vi "Get Cluster Elements (data types).vi"(8 "Error In":errorcluster, 9 "Type In":variant, 10 "Cluster":variant, 11 "Type Enum (Cluster)":T1=enum."Cluster") -> (0 "Error Out":errorcluster, 1 "Types Out":variant[](array[variant]), 2 "Cluster Elements":variant[](array[variant]))   [LabVIEW 2020]
doc: "This VI was created for use with the Read/Write Cluster VIs. It breaks a cluster up into its individual elements and passes the elements out in an array of variants.\n\nFreeware from Moore Good Ideas, www.mooregoodideas.com. Do not remove this line."
uses:
  <vilib>/Utility/VariantDataType/Type.ctl
  <vilib>/Utility/Data Type/NI_Data Type.lvlib
  <vilib>/Utility/VariantDataType/VariantType.lvlib
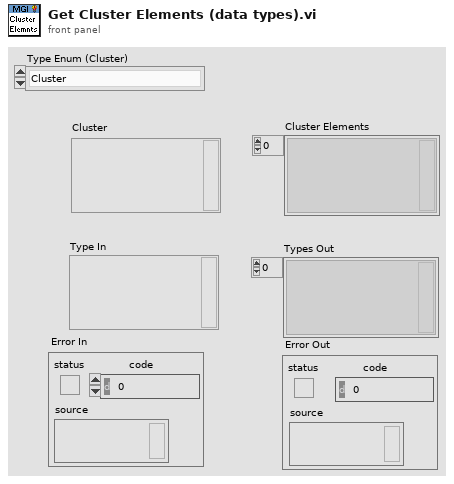
[diagram p1: front panel]
types:
  T1 = typedef "VariantType.lvlib/Type.ctl" = enum8{"Invalid Type", "Void", "I8", "I16", "I32", "I64", "U8", "U16", "U32", "U64", "Single Float", "Double Float", "Extended Float", "Single Complex", "Double Complex", "Extended Complex", "Enum U8", "Enum U16", "Enum U32", "Enum U64", "Single Float With Unit", "Double Float With Unit", "Extended Float With Unit", "Single Complex with Unit", "Double Complex with Unit", "Extended Complex with Unit", "Boolean", "String", "Path", "Picture", "Tag", "Array", "Cluster", "Variant", "LV Variant", "Waveform", "Timestamp", "Digital Waveform", "Digital Data", "ExpressData", "Refnum", "External Data", "VI", "Poly VI", "LabVIEW Class Instance", "Fixed Point"}
  T2 = typedef "NI_Data Type.lvlib/Data Type.ctl" = enum8{"Invalid Type", "Void", "I8", "I16", "I32", "I64", "U8", "U16", "U32", "U64", "Single Float", "Double Float", "Extended Float", "Single Complex", "Double Complex", "Extended Complex", "Enum U8", "Enum U16", "Enum U32", "Enum U64", "Single Float With Unit", "Double Float With Unit", "Extended Float With Unit", "Single Complex with Unit", "Double Complex with Unit", "Extended Complex with Unit", "Boolean", "String", "Path", "Picture", "Tag", "Array", "Cluster", "Variant", "LV Variant", "Waveform", "Timestamp", "Digital Waveform", "Digital Data", "ExpressData", "Refnum", "External Data", "VI", "Poly VI", "LabVIEW Class Instance", "Fixed Point", "Set Collection", "Map Collection"}
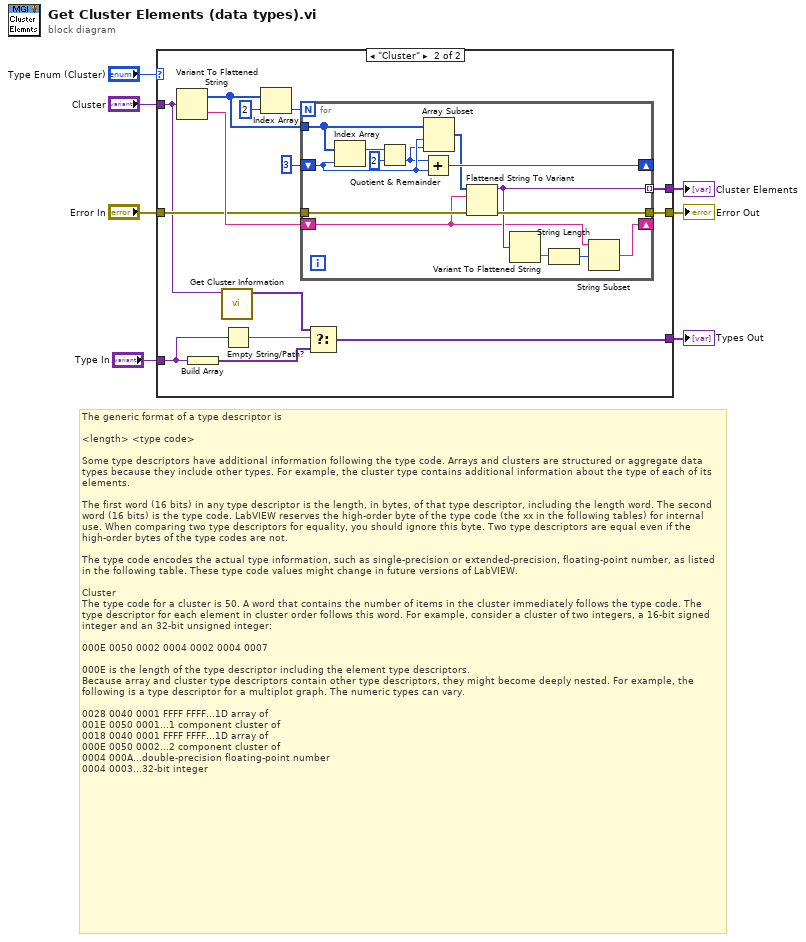
[diagram p0: block diagram]
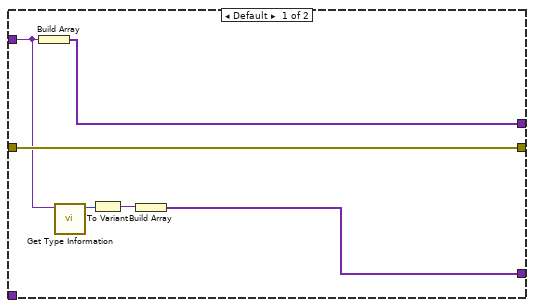
[diagram p2: hidden frame]
diagram:
  # "The generic format of a type descriptor is\n\n<length> <type code> \n\nSome type descriptors have additional information following the type code. Arrays and clusters are structured or aggregate data types because they include other types. For example, the cluster type contains additional information about the type of each of its elements.\n\nThe first word (16 bits) in any type descriptor is the length, in bytes, of that type descriptor, including the length word. The second word (16 bits) is the type code. LabVIEW reserves the high-order byte of the type code (the xx in the following tables) for internal use. When comparing two type descriptors for equality, you should ignore this byte. Two type descriptors are equal even if the high-order bytes of the type codes are not.\n\nThe type code encodes the actual type information, such as single-precision or extended-precision, floating-point number, as listed in the following table. These type code values might change in future versions of LabVIEW.\n\nCluster\nThe type code for a cluster is 50. A word that contains the number of items in the cluster immediately follows the type code. The type descriptor for each element in cluster order follows this word. For example, consider a cluster of two integers, a 16-bit signed integer and an 32-bit unsigned integer:\n\n000E 0050 0002 0004 0002 0004 0007 \n\n000E is the length of the type descriptor including the element type descriptors.\nBecause array and cluster type descriptors contain other type descriptors, they might become deeply nested. For example, the following is a type descriptor for a multiplot graph. The numeric types can vary.\n\n0028 0040 0001 FFFF FFFF...1D array of\n001E 0050 0001...1 component cluster of \n0018 0040 0001 FFFF FFFF...1D array of\n000E 0050 0002...2 component cluster of \n0004 000A...double-precision floating-point number \n0004 0003...32-bit integer"
  n1 = case shown="\"Cluster\"" "Type Enum (Cluster)" {
    tunnel: [w13 w21] -> w7
    tunnel: "Error In" -> [w13 w22]
    tunnel: "Cluster" -> [w11 w19]
    tunnel: [w12 w20] -> w3
    tunnel: "Type In" -> [_ w15]
    tunnel: [w8 w17] -> w1
    frame Default {
      n2 = Build Array(w11) -> (w12:variant[])
      n3 = call <vilib>:"Get Type Information.vi"("variant"=w11) -> ("type"=w10:T2)  [unwired: 6 in, 4 out]
      n4 = To Variant(anything=w10) -> (Variant=w9:variant)
      n5 = Build Array(w9) -> (w8:variant[])
    }
    frame "Cluster" {
      n6 = Variant To Flattened String(Variant=w19) -> (data string=w27:string, 1:w24:i16[])
      n7 = Build Array(w15) -> (w16:variant[])
      n8 = call <vilib>:"Get Cluster Information.vi"("variant"=w19) -> ("cluster elements"=w18:variant[])  [unwired: 9 in, 1 out]
      n9 = Empty String/Path?(string/path=w15) -> (empty?=w14:bool)
      n10 = Index Array(array=w24, index=2) -> (element=w26:i16)
      n11 = for {
        N: w26 -> [_]
        shift-right: [w40] -> _
        shift-left: 3 ("Index") -> [w39]
        tunnel: w24 -> [w41]
        tunnel: w22 -> [w34]
        tunnel: [w33] -> w21
        tunnel: [w31] -> w20 mode=indexing
        shift-right: [w29] -> _
        shift-left: w27 -> [w28]
        n12 = Index Array(array=w41, index=w39) -> (element=w37:i16)
        n13 = Quotient & Remainder(x=w37, y=i16 2) -> (floor(x/y)=w38:i16)  [unwired: 1 out]
        n14 = Add(x=w38, y=w39) -> (x+y=w40:i32)
        n15 = Array Subset(array=w41, index=w39, length=w38) -> (w35:i16[])
        n16 = Flattened String To Variant(4:w34, 6:w28, 7:w35) -> (0:w33:errorcluster, 3:w31:variant)
        n17 = Variant To Flattened String(Variant=w31) -> (data string=w32:string)  [unwired: 1 out]
        n18 = String Length(string=w32) -> (length=w30:i32)
        n19 = String Subset(string=w28, offset (0)=w30) -> (substring=w29:string)  [unwired: 1 in]
      }
      n20 = Select(t=w18, s=w14, f=w16) -> (s? t:f=w17:variant[])
    }
  }
  "Error Out" <- w7
  "Cluster Elements" <- w3
  "Types Out" <- w1
